vi "read_canvas.vi"() -> (1 "C 1":dbl, 2 "C 2":dbl, 3 "C 3":dbl, 4 "C 4":dbl, 6 "B 4":dbl, 7 "D 1":dbl, 8 "B 3":dbl, 9 "D 2":dbl, 10 "B 2":dbl, 11 "D 3":dbl, 12 "B 1":dbl, 13 "D 4":dbl, 15 "A 4":dbl, 16 "A 3":dbl, 17 "A 2":dbl, 18 "A 1":dbl)   [LabVIEW 2016]
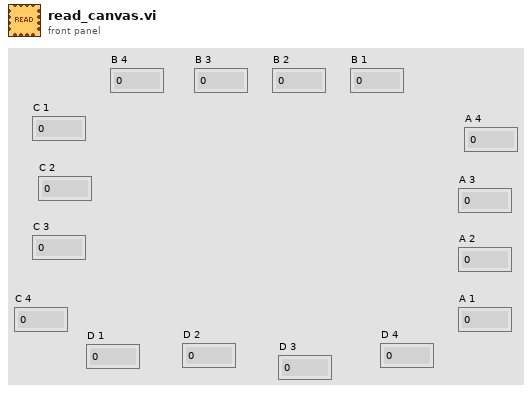
[diagram p1: front panel]
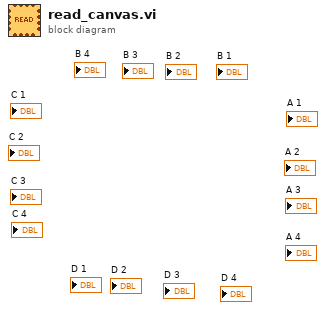
[diagram p0: block diagram]
diagram:
